vi "Acquire Comparison.vi"() -> ()   [LabVIEW 2013]
uses:
  lightfield-automation-labview/LightField Automation.lvclass
panel:
  in  "ExperimentName":string
  in  "Acquire":bool
  out "Acquire ROI 1, Frame 1, Row 1":dbl[](graph)
  out "Capture ROI 1, Frame 1, Row 1":dbl[](graph)
  in  "Capture":bool
  out "Acquire ROI 1, Frame 1":dbl[][](graph)
  out "Capture ROI 1, Frame 1":dbl[][](graph)
  in  "?":bool
  out "Exposures Per Frame":i32
  in  "Exposures Per Frame":i32=1
  out "Number of Frames":i32
  in  "Number of Frames":i32=1
  out "Exposure Time (s)":dbl
  in  "Exposure Time (s)":dbl=0.1
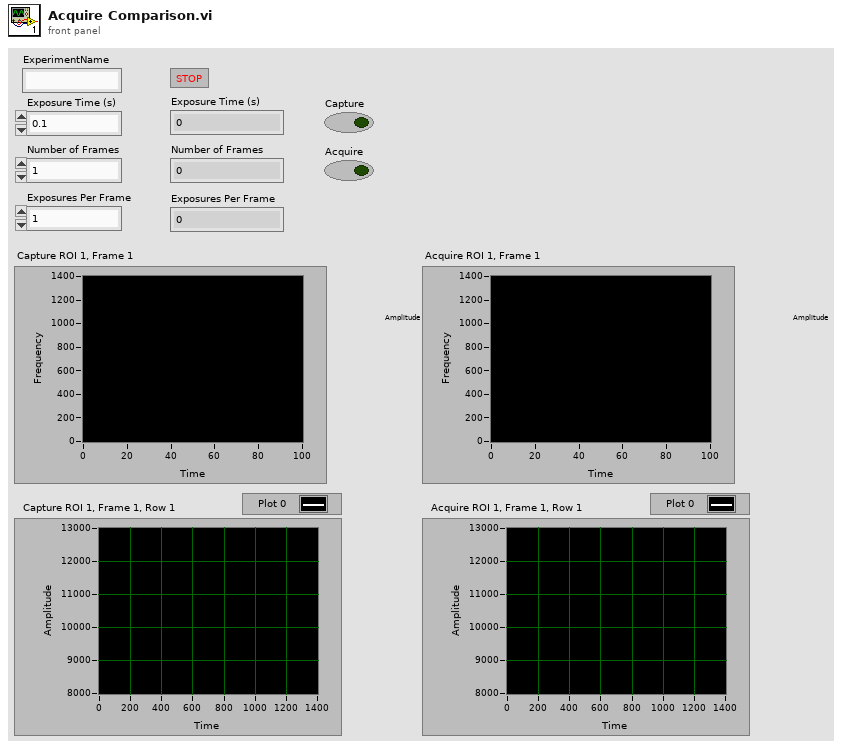
[diagram p1: front panel]
types:
  T1 = cluster{"Image":dbl[][][], "Frame Size":cluster{"F":i32, "Y":i32, "X":i32}}[]
  T2 = cluster{"Image":dbl[][][], "Frame Size":cluster{"F":i32, "Y":i32, "X":i32}}
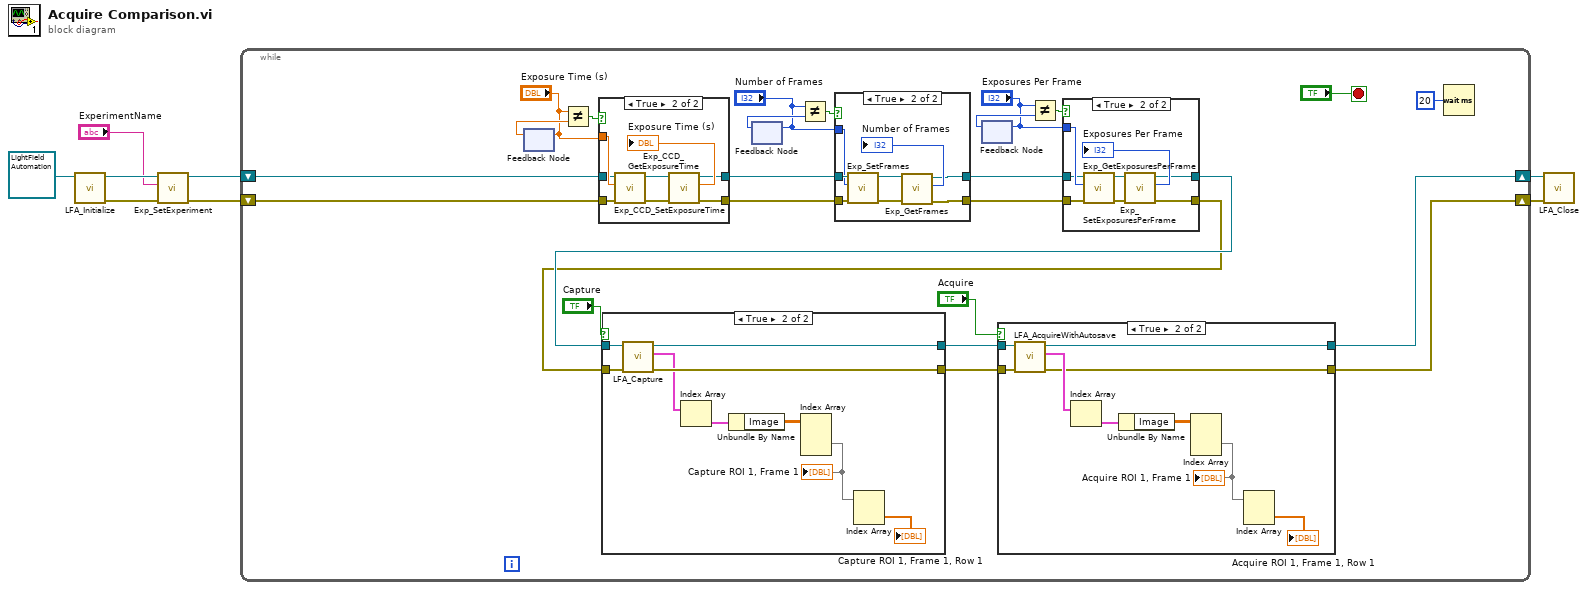
[diagram p0: block diagram]
diagram:
  n1 = call "LFA_Initialize.vi"("LightField Automation in"=refnum<class "LightField Automation.lvclass"> refnum ("LightField Automation.lvclass")) -> ("error out"=w6:errorcluster, "LightField Automation out"=w7:refnum<class "LightField Automation.lvclass">)  [unwired: 9 in]
  n2 = call "Exp_SetExperiment.vi"("error in (no error)"=w6, "ExperimentName"="ExperimentName", "LightField Automation in"=w7) -> ("error out"=w4:errorcluster, "LightField Automation out"=w3:refnum<class "LightField Automation.lvclass">)  [unwired: 7 in]
  n3 = while {
    shift-right: [w13] -> w1
    shift-left: w3 -> [w9]
    shift-right: [w12] -> w2
    shift-left: w4 -> [w10]
    stop <- "?" stop-if-true
    n4 = feedback-in #1("Exposure Time (s)") -> ()
    n5 = feedback #1() -> (w30:dbl)  [unwired: 1 in]
    n6 = Not Equal?(x="Exposure Time (s)", y=w30) -> (x != y?=w31:bool)
    n7 = case shown="True" w31 {
      tunnel: "Exposure Time (s)" -> [_ w82]
      tunnel: w9 -> [w76 w81]
      tunnel: w10 -> [w77 w80]
      tunnel: [w76 w79] -> w28
      tunnel: [w77 w78] -> w27
      frame False {
      }
      frame True {
        n8 = call "Exp_CCD_SetExposureTime.vi"("error in (no error)"=w80, "Exposure Time (s)"=w82, "LightField Automation in"=w81) -> ("error out"=w83:errorcluster, "LightField Automation out"=w84:refnum<class "LightField Automation.lvclass">)  [unwired: 7 in]
        n9 = call "Exp_CCD_GetExposureTime.vi"("error in (no error)"=w83, "LightField Automation in"=w84) -> ("error out"=w78:errorcluster, "Exposure Time (s)"=→"Exposure Time (s)":dbl, "LightField Automation out"=w79:refnum<class "LightField Automation.lvclass">)  [unwired: 7 in]
      }
    }
    n10 = feedback #2() -> (w26:i32)  [unwired: 1 in]
    n11 = feedback-in #2("Number of Frames") -> ()
    n12 = Not Equal?(x="Number of Frames", y=w26) -> (x != y?=w25:bool)
    n13 = case shown="True" w25 {
      tunnel: w28 -> [w67 w72]
      tunnel: w27 -> [w66 w71]
      tunnel: "Number of Frames" -> [_ w70]
      tunnel: [w67 w69] -> w20
      tunnel: [w66 w68] -> w19
      frame False {
      }
      frame True {
        n14 = call "Exp_SetFrames.vi"("error in (no error)"=w71, "Number of Frames"=w70, "LightField Automation in"=w72) -> ("error out"=w74:errorcluster, "LightField Automation out"=w75:refnum<class "LightField Automation.lvclass">)  [unwired: 7 in]
        n15 = call "Exp_GetFrames.vi"("error in (no error)"=w74, "LightField Automation in"=w75) -> ("error out"=w68:errorcluster, "Frames"=→"Number of Frames":i32, "LightField Automation out"=w69:refnum<class "LightField Automation.lvclass">)  [unwired: 7 in]
      }
    }
    n16 = feedback #3() -> (w23:i32)  [unwired: 1 in]
    n17 = feedback-in #3("Exposures Per Frame") -> ()
    n18 = Not Equal?(x="Exposures Per Frame", y=w23) -> (x != y?=w22:bool)
    n19 = case shown="True" w22 {
      tunnel: "Exposures Per Frame" -> [_ w62]
      tunnel: w20 -> [w57 w61]
      tunnel: w19 -> [w56 w60]
      tunnel: [w56 w59] -> w16
      tunnel: [w57 w58] -> w18
      frame False {
      }
      frame True {
        n20 = call "Exp_SetExposuresPerFrame.vi"("error in (no error)"=w60, "Exposures Per Frame"=w62, "LightField Automation in"=w61) -> ("error out"=w65:errorcluster, "LightField Automation out"=w64:refnum<class "LightField Automation.lvclass">)  [unwired: 7 in]
        n21 = call "Exp_GetExposuresPerFrame.vi"("error in (no error)"=w65, "LightField Automation in"=w64) -> ("error out"=w59:errorcluster, "Exposures Per Frame"=→"Exposures Per Frame":i32, "LightField Automation out"=w58:refnum<class "LightField Automation.lvclass">)  [unwired: 7 in]
      }
    }
    n22 = case shown="True" "Capture" {
      tunnel: w18 -> [w46 w48]
      tunnel: w16 -> [w45 w47]
      tunnel: [w46 w50] -> w15
      tunnel: [w45 w51] -> w14
      frame False {
      }
      frame True {
        n23 = call "LFA_Capture.vi"("error in (no error)"=w47, "LightField Automation in"=w48) -> ("error out"=w51:errorcluster, "Data"=w49:T1, "LightField Automation out"=w50:refnum<class "LightField Automation.lvclass">)  [unwired: 7 in]
        n24 = Index Array(array=w49) -> (element=w55:T2)  [unwired: 1 in]
        n25 = Unbundle By Name(w55) -> ("Image"=w54:dbl[][][])
        n26 = Index Array(array=w54) -> (element=w53:dbl[][])  [unwired: 3 in]
        "Capture ROI 1, Frame 1" <- w53
        n27 = Index Array(array=w53) -> (element=→"Capture ROI 1, Frame 1, Row 1":dbl[])  [unwired: 2 in]
      }
    }
    n28 = case shown="True" "Acquire" {
      tunnel: w15 -> [w35 w39]
      tunnel: w14 -> [w34 w40]
      tunnel: [w35 w38] -> w13
      tunnel: [w34 w36] -> w12
      frame False {
      }
      frame True {
        n29 = call "LFA_AcquireWithAutosave.vi"("error in (no error)"=w40, "LightField Automation in"=w39) -> ("error out"=w36:errorcluster, "Data"=w37:T1, "LightField Automation out"=w38:refnum<class "LightField Automation.lvclass">)  [unwired: 7 in]
        n30 = Index Array(array=w37) -> (element=w44:T2)  [unwired: 1 in]
        n31 = Unbundle By Name(w44) -> ("Image"=w43:dbl[][][])
        n32 = Index Array(array=w43) -> (element=w41:dbl[][])  [unwired: 3 in]
        "Acquire ROI 1, Frame 1" <- w41
        n33 = Index Array(array=w41) -> (element=→"Acquire ROI 1, Frame 1, Row 1":dbl[])  [unwired: 2 in]
      }
    }
    n34 = Wait (ms)(milliseconds to wait=u32 20) -> ()  [unwired: 1 out]
  }
  n35 = call "LFA_Close.vi"("error in (no error)"=w2, "LightField Automation in"=w1) -> ()  [unwired: 8 in, 2 out]
